vi "write_vector.vi"(1 "error in (no error)":errorcluster, 2 "1D data":dbl[](array[numeric]), 3 "file path (dialog if empty)":path) -> (0 "error out":errorcluster)   [LabVIEW 2021]
uses:
  <vilib>/Utility/file.llb/Write Delimited Spreadsheet (DBL).vi
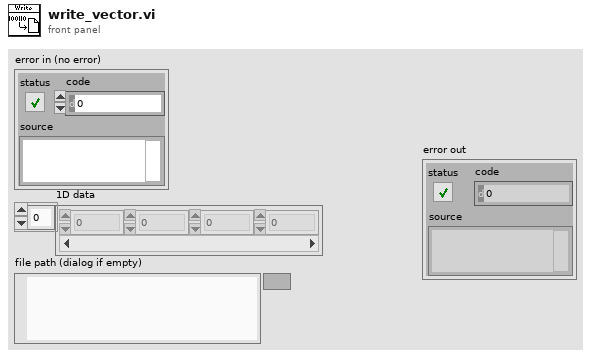
[diagram p1: front panel]
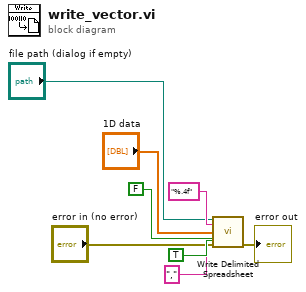
[diagram p0: block diagram]
diagram:
  n1 = call-poly <vilib>:"Write Delimited Spreadsheet.vi"("file path (dialog if empty)"="file path (dialog if empty)", "format (%.3f)"="%.4f", "1D data"="1D data", "append to file? (new file:F)"=FALSE, "error in (no error)"="error in (no error)", "transpose? (no:F)"=TRUE, "delimiter (\\t)"="," ("delimiter (\\t)")) -> ("error out"=→"error out":errorcluster)  [unwired: 7 in, 1 out]
